vi "niDTS BT BDR Tx Test Configure.vi"(0 "Dummy Test Handle In":T9, 7 "BT BDR Parameters":T1={"Channel"=0, "Dut Tx Power (dBm)"=0.0, "Auto Level"=FALSE, "External Attenuation (dB)"=0.0, "BDR Packet type"=enum."DH1", "Payload Data"=enum."PN9", "Burst Sync"=enum."NONE", "Packet length (bytes)"=0, "BD ADDRESS"="", "Modulation Measurement"={"ModAcc Enable"=FALSE, "CFO Enable"=FALSE, "Character Select"=enum."DF1", "Averages"=0, "Averaging Mode"=enum."RMS", "Measurement Duration (Symbols)"=0, "Measurement Offset (Symbols)"=0}, "Trace Enable"=FALSE, "OBW Measurement"={"OBW Enable"=FALSE, "OBW Averages"=0, "Averaging Type"=enum."RMS", "Measurement Interval Mode"=enum."AUTO", "Measurement Interval Length (sec)"=0.0}, "TXP Measurement"={"TXP Power Enable"=FALSE, "TXP Averages"=0, "Averaging Type"=enum."RMS"}, "IBE Measurement"={"IBE Enable"=FALSE, "IBE Averages"=164, "Averaging Type"=enum."LOG", "Numbe of Channels"=12329017, "Channel Mode"=enum."InBand", "Measurement Interval Mode"=enum."AUTO", "Measurement Interval Length (sec)"=0.0}, "Trigger"={"MinQuietTimeDuration (sec)"=0.0, "TriggerDelay (sec)"=0.0, "TriggerEdge"=enum."RISing", "TriggerSource"=enum."IMMediate", "TriggerThreshold (dB)"=0.0, "TriggerTimeout (sec)"=0.0}} {"Trigger"."MinQuietTimeDuration (sec)" format="%#_6p"}, 9 "ResultsIndex":u8=1, 11 "error in (no error)":errorcluster) -> (4 "Dummy Test Handle Out":T9, 15 "error out":errorcluster)   [LabVIEW 2014, in "niDTS BT.lvlib"]
uses:
  niDTS BT.lvlib
  Tx Test/Includes/niDTS BT Tx Test INC Handle.ctl
  Tx Test/Objects/BASE_class/niDTS BT Tx Test.lvclass
  Includes/niDTS BT BDR Tx Test INC Parameters.ctl
  Includes/niDTS BT INC BDR Packet Type.ctl
  Tx Test/Includes/niDTS BT Tx Test INC BD Payload Data.ctl
  Tx Test/Includes/niDTS BT Tx Test INC Modulation Characteristics.ctl
  Includes/niDTS BT INC OBW Measurement Parameters.ctl
  Includes/niDTS BT INC TXP Measurement Parameters.ctl
  Includes/niDTS BT INC BDR ACP Measurement Parameters.ctl
  Includes/niDTS BT DUT INC Trigger.ctl
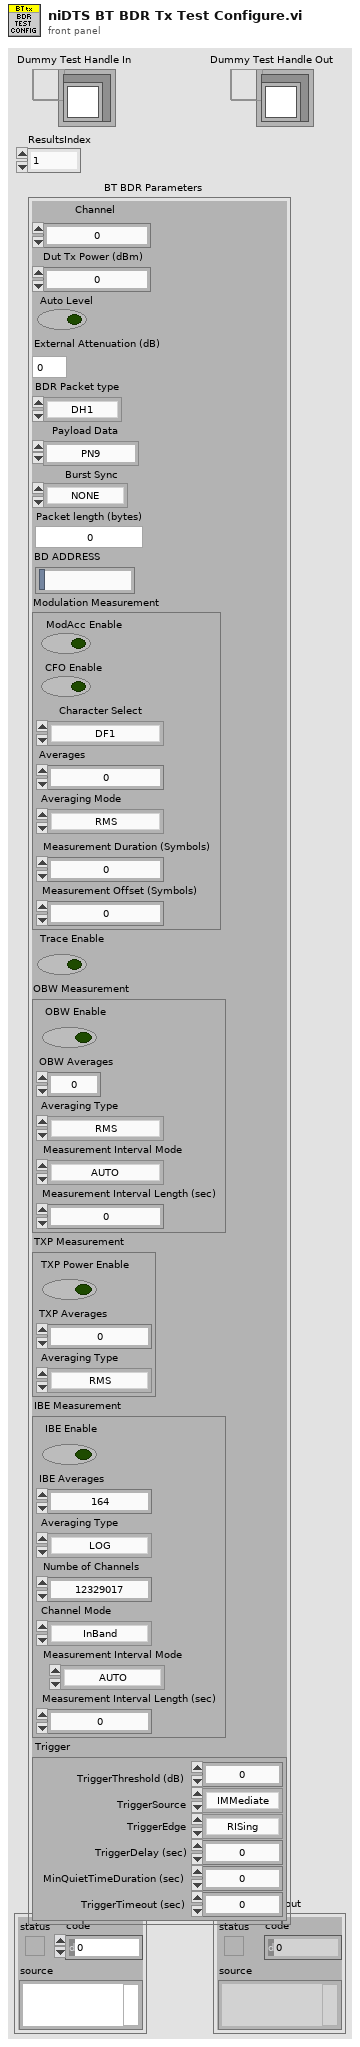
[diagram p1: front panel]
types:
  T1 = typedef "niDTS BT.lvlib/niDTS BT BDR Tx Test INC Parameters.ctl" = cluster{"Channel":i32, "Dut Tx Power (dBm)":dbl, "Auto Level":bool, "External Attenuation (dB)":dbl, "BDR Packet type":T2, "Payload Data":T3, "Burst Sync":enum16{"NONE", "PREamble"}, "Packet length (bytes)":i32, "BD ADDRESS":string, "Modulation Measurement":cluster{"ModAcc Enable":bool, "CFO Enable":bool, "Character Select":T4, "Averages":i32, "Averaging Mode":enum16{"RMS", "LOG", "SCALAR", "MAX", "MIN", "VECTOR"}, "Measurement Duration (Symbols)":i32, "Measurement Offset (Symbols)":i32}, "Trace Enable":bool, "OBW Measurement":T5, "TXP Measurement":T6, "IBE Measurement":T7, "Trigger":T8}
  T2 = typedef "niDTS BT.lvlib/niDTS BT INC BDR Packet Type.ctl" = enum16{"NULL", "POLL", "FHS", "DM1", "DH1", "HV1", "HV2", "HV3", "EV3", "DV", "AUX1", "DM3", "DH3", "EV4", "EV5", "DM5", "DH5"}
  T3 = typedef "niDTS BT.lvlib/niDTS BT Tx Test INC BD Payload Data.ctl" = enum16{"0", "1", "01", "00001111", "PN9", "AUTO"}
  T4 = typedef "niDTS BT.lvlib/niDTS BT Tx Test INC Modulation Characteristics.ctl" = enum16{"DF1", "DF2", "BOTH"}
  T5 = typedef "niDTS BT.lvlib/niDTS BT INC OBW Measurement Parameters.ctl" = cluster{"OBW Enable":bool, "OBW Averages":i32, "Averaging Type":enum16{"RMS", "LOG", "SCALAR", "MAX", "MIN", "VECTOR"}, "Measurement Interval Mode":enum16{"AUTO", "MANUAL"}, "Measurement Interval Length (sec)":dbl}
  T6 = typedef "niDTS BT.lvlib/niDTS BT INC TXP Measurement Parameters.ctl" = cluster{"TXP Power Enable":bool, "TXP Averages":i32, "Averaging Type":enum16{"RMS", "LOG", "SCALAR", "MAX", "MIN"}}
  T7 = typedef "niDTS BT.lvlib/niDTS BT INC BDR ACP Measurement Parameters.ctl" = cluster{"IBE Enable":bool, "IBE Averages":i32, "Averaging Type":enum16{"RMS", "LOG", "SCALAR", "MAX", "MIN", "VECTOR"}, "Numbe of Channels":i32, "Channel Mode":enum16{"InBand", "Centered"}, "Measurement Interval Mode":enum16{"AUTO", "MANUAL"}, "Measurement Interval Length (sec)":dbl}
  T8 = typedef "niDTS BT.lvlib/niDTS BT DUT INC Trigger.ctl" = cluster{"MinQuietTimeDuration (sec)":dbl, "TriggerDelay (sec)":dbl, "TriggerEdge":enum16{"RISing", "FALLing"}, "TriggerSource":enum16{"IMMediate", "RF0", "PFI0", "PFI1", "RTS0", "RTS1", "RTS2", "RTS3", "RTS4", "RTS5", "RTS6", "RTS7", "PXIStar", "SOFT"}, "TriggerThreshold (dB)":dbl, "TriggerTimeout (sec)":dbl}
  T9 = typedef "niDTS BT.lvlib/niDTS BT Tx Test INC Handle.ctl" = refnum<data-value>
  T10 = typedef "niDTS BT.lvlib/niDTS BT Tx Test INC Parameters.ctl" = cluster{"Channel":i32, "Data Rate ":i32, "Dut Tx Power":dbl, "External Attenuation (dB)":dbl[], "Auto Level":bool, "Packet type":T11, "Payload Pattern":T3, "Burst Sync":enum16{"NONE", "PREamble"}, "BD ADDRESS":u32, "Packet Length, bytes":i32, "ModAcc Measurement Paramaters":cluster{"ModAcc Enable":bool, "CFO Enable":bool, "Character Select":T4, "Averages":i32, "Averaging Mode":enum16{"RMS", "LOG", "SCALAR", "MAX", "MIN", "VECTOR"}, "Measurement Length":i32, "Measurement Offset":i32}, "OBW Measurement Parameters":T5, "TXP Measurement Parameters":T6, "IBE  Measurement Parameters":T12, "Trace Enable":bool, "Trigger":T8}
  T11 = typedef "niDTS BT.lvlib/niDTS BT INC Packet Type.ctl" = enum16{"NULL", "POLL", "FHS", "DM1", "DH1", "HV1", "HV2", "HV3", "EV3", "DV", "AUX1", "DM3", "DH3", "EV4", "EV5", "DM5", "DH5", "LE-TP"}
  T12 = typedef "niDTS BT.lvlib/niDTS BT INC EDR IBE Measurement Parameters.ctl" = cluster{"IBE Enable":bool, "IBE Averages":i32, "Averaging Type":enum16{"RMS", "LOG", "SCALAR", "MAX", "MIN", "VECTOR"}, "Numbe of Channels":i32, "Channel Mode":enum16{"InBand", "Centered"}, "Measurement Interval Mode":enum16{"AUTO", "MANUAL"}, "Measurement Interval Length (sec)":dbl}
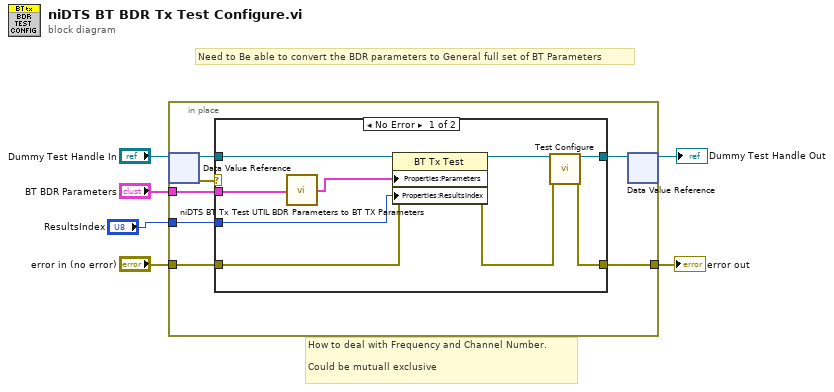
[diagram p0: block diagram]
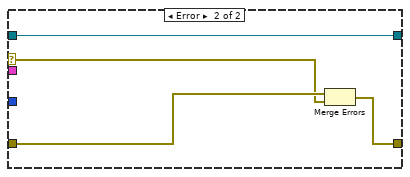
[diagram p2: hidden frame]
diagram:
  # "Need to Be able to convert the BDR parameters to General full set of BT Parameters"
  # "How to deal with Frequency and Channel Number.\n\nCould be mutuall exclusive"
  n1 = in-place {
    in-place-border: "error in (no error)" -> [w10]
    in-place-border: [w9] -> w5
    in-place-border: "BT BDR Parameters" -> [w8]
    in-place-border: "ResultsIndex" -> [w7]
    n2 = in-place-dvr #1("Dummy Test Handle In") -> (w12:refnum<class "niDTS BT Tx Test.lvclass">, w13:errorcluster)
    n3 = case shown="No Error" w13 {
      selector: w13 -> [_ w24]
      tunnel: w12 -> [w22 w26]
      tunnel: [w18 w26] -> w11
      tunnel: w10 -> [w21 w25]
      tunnel: [w19 w23] -> w9
      tunnel: w8 -> [w15 _]
      tunnel: w7 -> [w14 _]
      frame No Error {
        n4 = call "niDTS BT Tx Test UTIL BDR Parameters to BT TX Parameters.vi"("BT BDR Parameters"=w15) -> ("BT Tx Parameters"=w16:T10)  [unwired: 14 in]
        n5 = property class="BT Tx Test"(reference=w22, error in=w21, "Properties:Parameters"=w16, "Properties:ResultsIndex"=w14) -> (reference out=w17:refnum<class "niDTS BT Tx Test.lvclass">, error out=w20:errorcluster)
        n6 = call-dynamic "Test Configure.vi"("Template Tx Test in"=w17, "error in (no error)"=w20) -> ("Template Tx Test out"=w18:refnum<class "niDTS BT Tx Test.lvclass">, "error out"=w19:errorcluster)  [unwired: 12 in]
      }
      frame Error {
        n7 = Merge Errors(w25, w24) -> (w23:errorcluster)
      }
    }
    n8 = in-place-dvr #1(w11) -> (→"Dummy Test Handle Out":T9)  [unwired: 1 out]
  }
  "error out" <- w5
